vi "KeyChange.vi"(9 "新键名":string, 10 "原键名":string, 11 "段名":string) -> ()   [LabVIEW 2018]
uses:
  <vilib>/Utility/config.llb/Read Key (String).vi
  <vilib>/Utility/config.llb/Write Key (String).vi
  <vilib>/Utility/config.llb/NI_LVConfig.lvlib
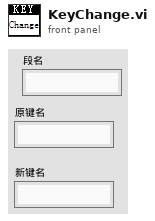
[diagram p1: front panel]
types:
  T1 = typedef "NI_LVConfig.lvlib/Config Data RefNum.ctl" = refnum<k1>
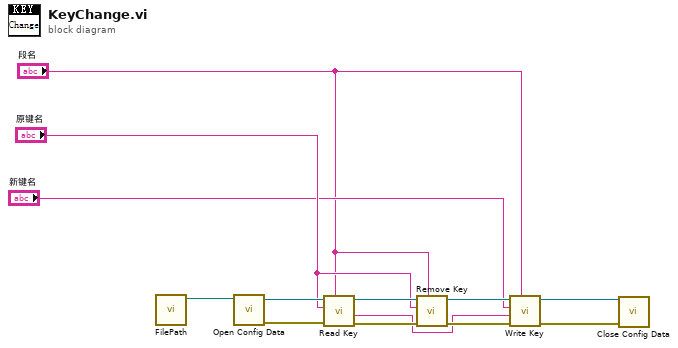
[diagram p0: block diagram]
diagram:
  n1 = call "FilePath.vi"() -> ("添加的路径"=w13:path)  [unwired: 11 in]
  n2 = call <vilib>:"Open Config Data.vi"("configuration file path"=w13) -> ("error out"=w11:errorcluster, "refnum"=w12:T1)  [unwired: 8 in, 1 out]
  n3 = call-poly <vilib>:"Read Key.vi"("section"="段名", "error in (no error)"=w11, "key"="原键名", "refnum"=w12) -> ("error out"=w9:errorcluster, "value"=w5:string, "refnum out"=w10:T1)  [unwired: 4 in, 1 out]
  n4 = call <vilib>:"Remove Key.vi"("section"="段名", "error in (no error)"=w9, "key"="原键名", "refnum"=w10) -> ("error out"=w6:errorcluster, "refnum out"=w7:T1)  [unwired: 5 in, 1 out]
  n5 = call-poly <vilib>:"Write Key.vi"("section"="段名", "error in (no error)"=w6, "value"=w5, "key"="新键名", "refnum"=w7) -> ("error out"=w1:errorcluster, "refnum out"=w2:T1)  [unwired: 4 in, 1 out]
  n6 = call <vilib>:"Close Config Data.vi"("error in (no error)"=w1, "refnum"=w2) -> ()  [unwired: 8 in, 2 out]
